vi "Identify.vi"(8 "error in (no error)":errorcluster, 11 "TXT in":refnum<class "TXT.lvclass">=refnum) -> (0 "error out":errorcluster, 2 "Boolean":bool, 3 "TXT out":refnum<class "TXT.lvclass">)   [LabVIEW 2016, in "TXT.lvclass"]
uses:
  TXT.lvclass
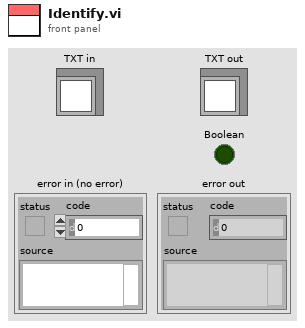
[diagram p1: front panel]
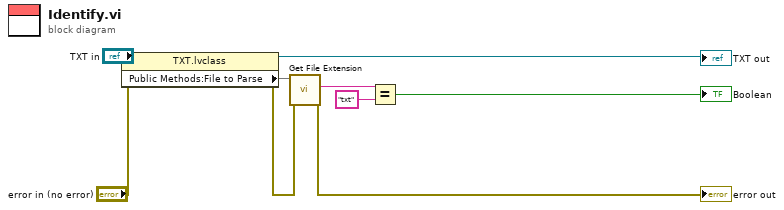
[diagram p0: block diagram]
diagram:
  n1 = property class="TXT.lvclass"(reference="TXT in", error in="error in (no error)") -> (reference out=→"TXT out":refnum<class "TXT.lvclass">, error out=w5:errorcluster, "Public Methods:File to Parse"=w6)
  n2 = call <vilib>:"Get File Extension.vi"("error in (no error)"=w5, "file"=w6) -> ("error out"=→"error out":errorcluster, "lowercase file extension"=w3:string)  [unwired: 5 in, 3 out]
  n3 = Equal?(x=w3, y="txt") -> (x = y?=→"Boolean":bool)
